vi "Character Count Limit Exceeded.vi"(10 "Response String in":string, 11 "Character Count Limit":i32) -> (2 "Limit Exceeded":bool)   [LabVIEW 2017, in "SSH.lvlib"]
doc: "Tests if the character limit count has been exceeded (ignores a value of 0)"
uses:
  SSH.lvlib
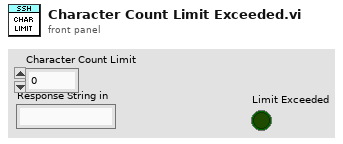
[diagram p1: front panel]
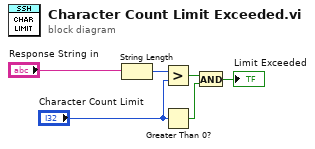
[diagram p0: block diagram]
diagram:
  n1 = String Length(string="Response String in") -> (length=w5:i32)
  n2 = Greater?(x=w5, y="Character Count Limit") -> (0:w3:bool)
  n3 = Greater Than 0?(x="Character Count Limit") -> (x > 0?=w2:bool)
  n4 = And(x=w3, y=w2) -> (x .and. y?=→"Limit Exceeded":bool)
